vi "Or_all_Errors.vi"(10 "Alarms in":T1, 11 "Alarms in 2":T1) -> (3 "Alarms out":T1)   [LabVIEW 2018]
uses:
  Controls/Clusts/DigOutClust.ctl
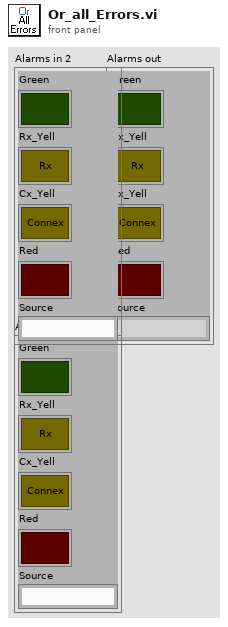
[diagram p1: front panel]
types:
  T1 = typedef "DigOutClust.ctl" = cluster{"Green":bool, "Rx_Yell":bool, "Cx_Yell":bool, "Red":bool, "Source":string}
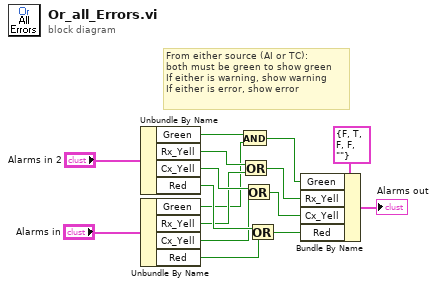
[diagram p0: block diagram]
diagram:
  # "From either source (AI or TC):\nboth must be green to show green\nIf either is warning, show warning\nIf either is error, show error"
  n1 = Unbundle By Name("Alarms in 2") -> ("Green"=w3:bool, "Rx_Yell"=w6:bool, "Cx_Yell"=w8:bool, "Red"=w10:bool)
  n2 = Unbundle By Name("Alarms in") -> ("Green"=w2:bool, "Rx_Yell"=w7:bool, "Cx_Yell"=w9:bool, "Red"=w11:bool)
  n3 = And(x=w3, y=w2) -> (x .and. y?=w1:bool)
  n4 = Or(x=w6, y=w7) -> (x .or. y?=w13:bool)
  n5 = Or(x=w8, y=w9) -> (x .or. y?=w14:bool)
  n6 = Or(x=w10, y=w11) -> (x .or. y?=w15:bool)
  n7 = Bundle By Name(cluster=T1 {"Green"=FALSE, "Rx_Yell"=TRUE, "Cx_Yell"=FALSE, "Red"=FALSE, "Source"=""} ("Alarms"), "Green"=w1, "Rx_Yell"=w13, "Cx_Yell"=w14, "Red"=w15) -> (→"Alarms out":T1)
